vi "Configure User Compensation.vi"(5 "Retry Attempts (0)":i32 min=0, 7 "Fast Comms (F)":bool, 8 "error in":errorcluster, 10 "Compensation (%)":dbl, 11 "VISA resource name":refnum<visa-resource-name>) -> (0 "error out":errorcluster, 2 "Response Compensation":dbl, 3 "VISA resource name out":refnum<visa-resource-name>)   [LabVIEW 2020, in "ChromTech MX-Class Drivers.lvlib"]
doc: "Stores the user flow rate compensation. Input range is 85.0 to 115.0 (i.e. +- 15.0 % compensation)."
uses:
  <instrlib>/RxnRover/ChromtechNextGenDriver/ChromTech MX-Class Drivers.lvlib
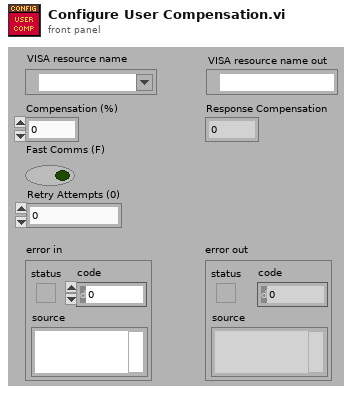
[diagram p1: front panel]
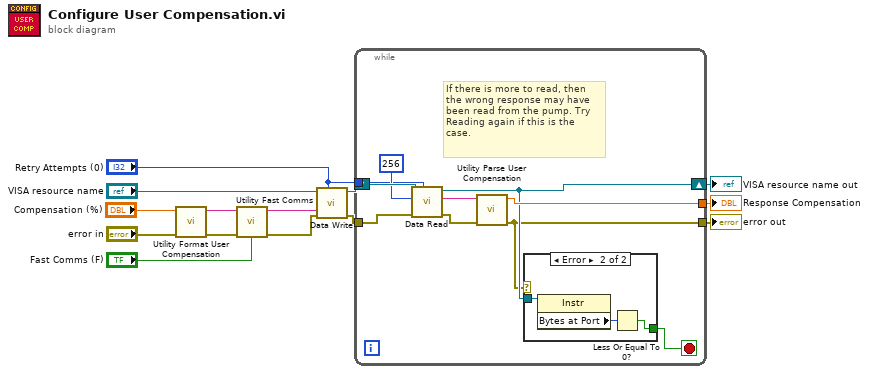
[diagram p0: block diagram]
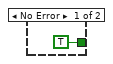
[diagram p2: hidden frame]
diagram:
  n1 = call <instrlib>:"Utility Format User Compensation.vi"("error in (no error)"="error in", "Compensation (%)"="Compensation (%)") -> ("error out"=w6:errorcluster, "Formatted Compensation"=w5:string)  [unwired: 8 in]
  n2 = call <instrlib>:"Utility Fast Comms.vi"("Fast Comms"="Fast Comms (F)", "Command"=w5) -> ("Fast Command"=w9:string)  [unwired: 9 in]
  n3 = call <instrlib>:"Data Write.vi"("Retry Attempts (0)"="Retry Attempts (0)", "error in (no error)"=w6, "Command"=w9, "VISA Refnum in"="VISA resource name") -> ("error out"=w11:errorcluster, "VISA Refnum out"=w12:refnum<visa-resource-name>)  [unwired: 6 in]
  n4 = while {
    tunnel: [w19] -> w10
    tunnel: "Retry Attempts (0)" -> [w17]
    shift-right: [w16] -> w2
    shift-left: w12 -> [w23]
    tunnel: w11 -> [w22]
    tunnel: [w15] -> w1
    stop <- w14 stop-if-true
    # "If there is more to read, then\nthe wrong response may have\nbeen read from the pump. Try\nReading again if this is the\ncase."
    n5 = call <instrlib>:"Data Read.vi"("Retry Attempts (0)"=w17, "error in (no error)"=w22, "Bytes to read"=256, "VISA Refnum in"=w23) -> ("error out"=w18:errorcluster, "read buffer"=w20:string, "VISA Refnum out"=w16:refnum<visa-resource-name>)  [unwired: 5 in]
    n6 = call <instrlib>:"Utility Parse User Compensation.vi"("error in (no error)"=w18, "Input String"=w20) -> ("error out"=w15:errorcluster, "Compensation"=w19:dbl)  [unwired: 8 in]
    n7 = case shown="Error" w15 {
      tunnel: w16 -> [_ w27]
      tunnel: [TRUE w25] -> w14
      frame No Error {
      }
      frame Error {
        n8 = property class="Instr"(reference=w27) -> ("Bytes at Port"=w26:u32)  [unwired: 1 in, 2 out]
        n9 = Less Or Equal To 0?(x=w26) -> (x <= 0?=w25:bool)
      }
    }
  }
  "VISA resource name out" <- w2
  "error out" <- w1
  "Response Compensation" <- w10
